vi "Get Value From DVR.vi"(8 "error in (no error)":errorcluster, 10 "DVR Ref in":refnum<vi>) -> (0 "error out":errorcluster, 2 "Controls[]":refnum<vi>[](array[refnum]))   [LabVIEW 2018]
uses:
  <vilib>/Utility/miscctls.llb/LVPointTypeDef.ctl
panel:
  in  "DVR in":refnum<data-value>
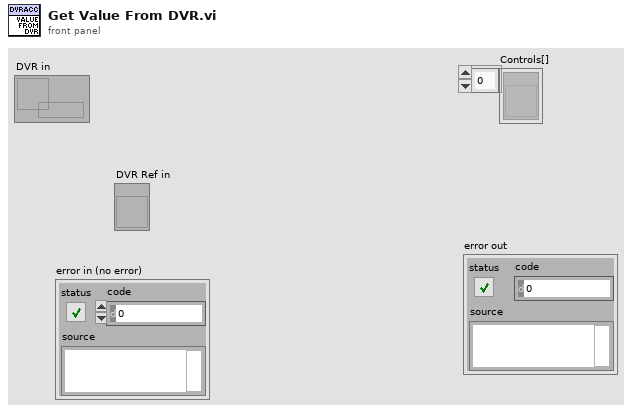
[diagram p1: front panel]
types:
  T1 = enum8{"Probe", "Diagram", "Panel Control", "3D Panel Control", "Dialog Panel Control", "Panel Indicator", "3D Panel Indicator", "Dialog Panel Indicator", "Power PC Control", "Power PC Indicator", "Silver Control", "Silver Indicator", "NXG Style Control", "NXG Style Indicator"}
  T2 = typedef "LVPointTypeDef.ctl" = cluster{"Horizontal":i16, "Vertical":i16}
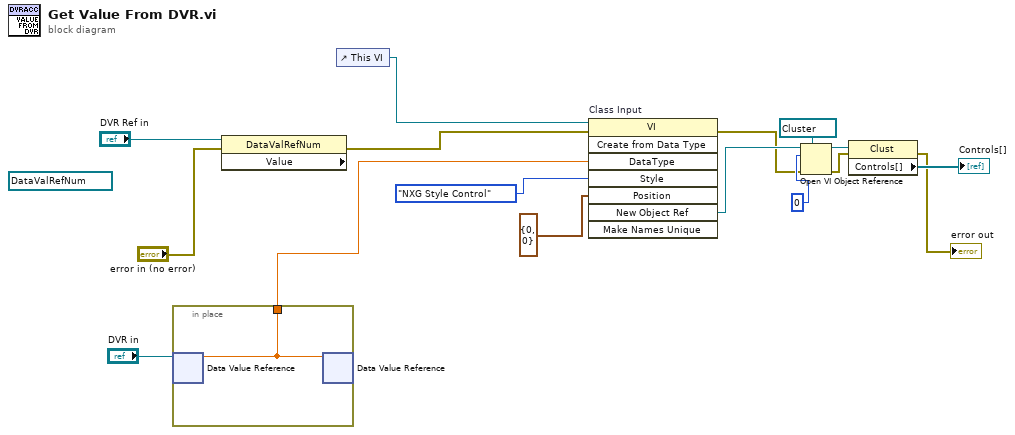
[diagram p0: block diagram]
diagram:
  (unwired) refnum<vi> refnum ("DataValRefNum in")
  n1 = in-place {
    in-place-border: [w17] -> w1
    n2 = in-place-dvr #1("DVR in") -> (w17:dbl)  [unwired: 1 out]
    n3 = in-place-dvr #1(w17) -> ()  [unwired: 2 out]
  }
  n4 = property class="DataValRefNum" props=["Value"](reference="DVR Ref in", error in="error in (no error)") -> (error out=w7:errorcluster)  [unwired: 2 out]
  n5 = control-ref of="This VI"() -> (w3:refnum<vi>)
  n6 = invoke on="Class Input" class="VI" method="Create from Data Type"(reference=w3, error in=w7, "DataType"=w1, "Style"=T1."NXG Style Control", "Position"=T2 {"Horizontal"=0, "Vertical"=0}) -> (error out=w6:errorcluster, "New Object Ref"=w9:refnum<vi>)  [unwired: 3 in, 6 out]
  n7 = Open VI Object Reference(7:refnum<vi> refnum ("Numeric"), 8:w6, 10:0, 11:w9) -> (0:w11:errorcluster, 3:w12:refnum<vi>)
  n8 = property class="Clust"(reference=w12, error in=w11) -> (error out=→"error out":errorcluster, "Controls[]"=→"Controls[]":refnum<vi>[])  [unwired: 1 out]
